vi "test_Send Data to FPGA.vi"(8 "error in (no error)":errorcluster, 11 "Data in":u64[](array[numeric])=[5631702913073631, 5629503829180420, 5629508124147720, 5629503829180426, 5629508124147722, 5629503829180426, 5629508124147722, 5629503829180426, 5629508124147722, 5631707147403291]) -> (0 "error out":errorcluster)   [LabVIEW 2016]
uses:
  Host/Typedefs/LV2G Operation.ctl
  Host/Typedefs/IO Buffer Operation.ctl
panel:
  out "Data out":u64[](array[numeric])=[5631702913073631, 5629503829180420, 5629508124147720, 5629503829180426, 5629508124147722, 5629503829180426, 5629508124147722, 5629503829180426, 5629508124147722, 5631707147403291]
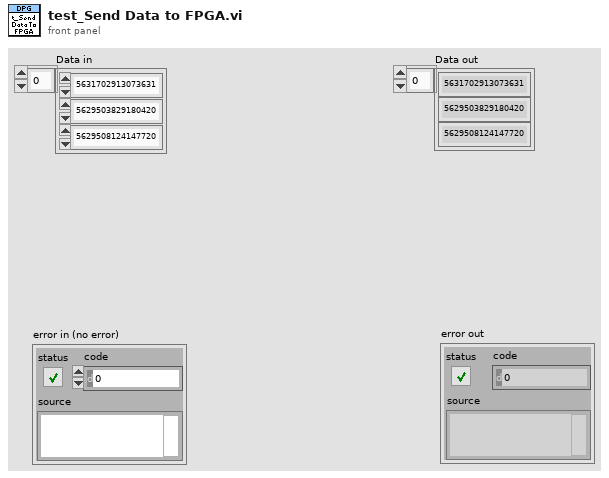
[diagram p1: front panel]
types:
  T1 = typedef "IO Buffer Operation.ctl" = enum16{"Initialize", "Write IO Data_Rd", "Read IO Data_Rd", "Write IO Data_Wr", "Read IO Data_Wr", "Write  IO Data_Dir", "Read  IO Data_Dir", "Write Host to Target FIFO", "Read Host to Target FIFO", "Write Target to Host FIFO", "Read Target to Host FIFO", "Write Monitor Enable?", "Read Monitor Enable?", "Close"}
  T2 = typedef "LV2G Operation.ctl" = enum16{"Initialize", "Set", "Get", "Close"}
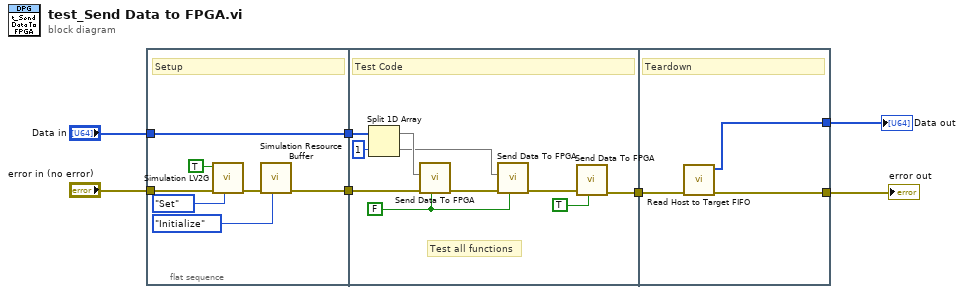
[diagram p0: block diagram]
diagram:
  n1 = flat-sequence {
    tunnel: "error in (no error)" -> [w14]
    tunnel: [w9] -> w7
    tunnel: "Data in" -> [w8]
    tunnel: [w8] -> w3
    tunnel: w7 -> [w19]
    tunnel: [w21] -> w6
    tunnel: w3 -> [w24]
    tunnel: [w26] -> w4
    tunnel: w6 -> [w27]
    tunnel: [w25] -> w2
    frame #0 {
      # "Setup"
      n2 = call "Simulation LV2G.vi"("Operation (Get)"=LV2G_Operation."Set", "error in (no error)"=w14, "Simulation?"=TRUE) -> ("error out"=w11:errorcluster)  [unwired: 7 in, 1 out]
      n3 = call "Simulation Resource Buffer.vi"("IO Buffer Operation"=IO_Buffer_Operation."Initialize", "error in (no error)"=w11) -> ("error out"=w9:errorcluster)  [unwired: 7 in, 2 out]
    }
    frame #1 {
      w17 = FALSE ("Write to FPGA(T)")
      # "Test all functions"
      # "Test Code"
      n4 = Split 1D Array(array=w24, index=1) -> (first subarray=w16:u64[], second subarray=w15:u64[])
      n5 = call "Send Data To FPGA.vi"("Write to FPGA(T)"=w17, "error in (no error)"=w19, "Data"=w16) -> ("error out"=w18:errorcluster)  [unwired: 7 in, 1 out]
      n6 = call "Send Data To FPGA.vi"("Write to FPGA(T)"=w17, "error in (no error)"=w18, "Data"=w15) -> ("error out"=w23:errorcluster)  [unwired: 7 in, 1 out]
      n7 = call "Send Data To FPGA.vi"("Write to FPGA(T)"=TRUE, "error in (no error)"=w23) -> ("error out"=w21:errorcluster)  [unwired: 8 in, 1 out]
    }
    frame #2 {
      # "Teardown"
      n8 = call "Read Host to Target FIFO.vi"("error in (no error)"=w27) -> ("error out"=w26:errorcluster, "Host to Target FIFO"=w25:u64[])  [unwired: 9 in]
    }
  }
  "error out" <- w4
  "Data out" <- w2
